vi "Write memory hierarchy.vi"(8 "error in (no error)":errorcluster, 10 "memory hierarchy":T1, 11 "CEF_HierarchyRepo in":refnum<class "CEF_HierarchyRepo.lvclass">) -> (0 "error out":errorcluster, 3 "CEF_HierarchyRepo out":refnum<class "CEF_HierarchyRepo.lvclass">)   [LabVIEW 2023, in "CEF.lvlib" / "CEF_HierarchyRepo.lvclass"]
uses:
  CEF_HierarchyRepo.lvclass
  memory hierarchy.ctl
  full hierarchy.ctl
  tree serializer/hierarchy element.ctl
  serializable configuration/CEF_serializable configuration.lvclass
  CEF_HierarchyRepo.lvclass/CEF_HierarchyRepo.ctl
  CEF.lvlib
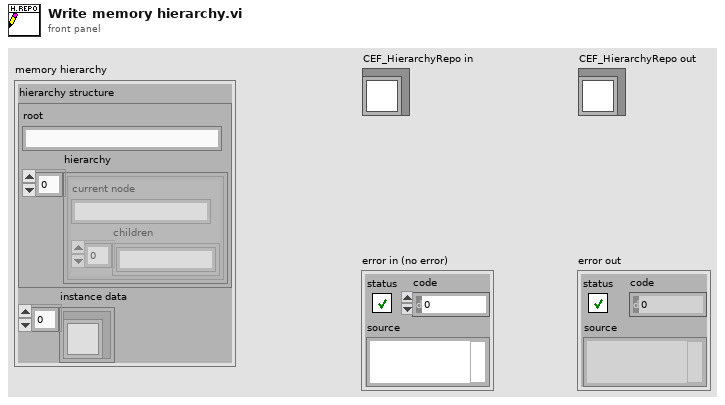
[diagram p1: front panel]
types:
  T1 = typedef "CEF.lvlib/CEF_HierarchyRepo.lvclass/memory hierarchy.ctl" = cluster{"hierarchy structure":T2, "instance data":refnum<class "CEF_serializable configuration.lvclass">[]}
  T2 = typedef "CEF.lvlib/CEF_HierarchyRepo.lvclass/full hierarchy.ctl" = cluster{"root":string, "hierarchy":T3[]}
  T3 = typedef "CEF.lvlib/hierarchy element.ctl" = cluster{"current node":string, "children":string[]}
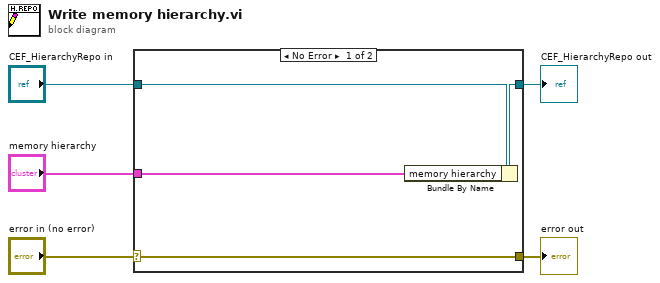
[diagram p0: block diagram]
diagram:
  n1 = case shown="No Error" "error in (no error)" {
    selector: "error in (no error)" -> [w9 w10]
    tunnel: [w9 w10] -> w4
    tunnel: [w7 w11] -> w2
    tunnel: "CEF_HierarchyRepo in" -> [w8 w11]
    tunnel: "memory hierarchy" -> [w6 _]
    frame No Error {
      n2 = Bundle By Name(cluster=w8, "memory hierarchy"=w6) -> (w7:refnum<class "CEF_HierarchyRepo.lvclass">)
    }
    frame Error {
    }
  }
  "error out" <- w4
  "CEF_HierarchyRepo out" <- w2
